vi "Create test signal.vi"(8 "Number of samples":dbl=10000.0, 10 "Downsample factor":i32, 11 "Sample rate":dbl) -> (1 "dt":dbl, 2 "signal out":waveform(dbl)={"t0"=timestamp(0.001 s since 1904-01-01), "dt"=1.0, "Y"=[]}, 3 "Y":fxp<+/-,16,14>[](array[numeric]))   [LabVIEW 2013]
uses:
  <vilib>/measure/NI_MABase.lvlib
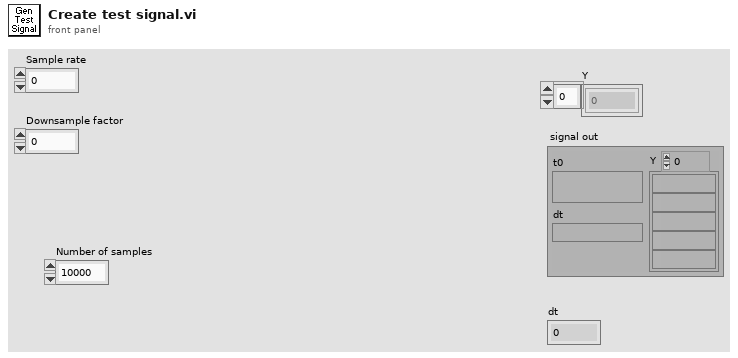
[diagram p1: front panel]
types:
  T1 = cluster{"frequency":dbl, "amplitude":dbl, "phase":dbl}
  T2 = cluster{"frequency":dbl, "amplitude":dbl, "phase":dbl}[]
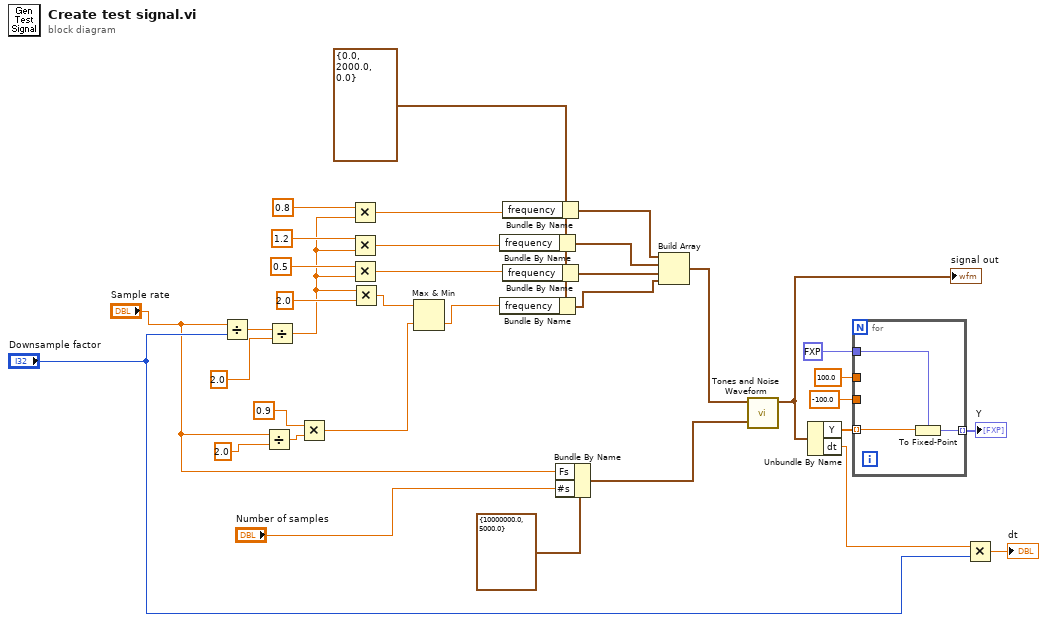
[diagram p0: block diagram]
diagram:
  w20 = T1 {"frequency"=0.0, "amplitude"=2000.0, "phase"=0.0} ("tone f, a, p")
  n1 = Divide(x="Sample rate", y="Downsample factor") -> (x/y=w28:dbl)
  n2 = Divide(x="Sample rate", y=2.0) -> (x/y=w5:dbl)
  n3 = Divide(x=w28, y=2.0) -> (x/y=w22:dbl)
  n4 = Multiply(x=0.9, y=w5) -> (x*y=w2:dbl)
  n5 = Multiply(x=0.8, y=w22) -> (x*y=w21:dbl)
  n6 = Multiply(x=1.2, y=w22) -> (x*y=w19:dbl)
  n7 = Multiply(x=0.5, y=w22) -> (x*y=w18:dbl)
  n8 = Multiply(x=w22, y=2.0 ("x")) -> (x*y=w3:dbl)
  n9 = Max & Min(x=w3, y=w2) -> (min(x,y)=w1:dbl)  [unwired: 1 out]
  n10 = Bundle By Name(cluster=w20, "frequency"=w19) -> (w16:T1)
  n11 = Bundle By Name(cluster=w20, "frequency"=w1) -> (w14:T1)
  n12 = Bundle By Name(cluster=w20, "frequency"=w21) -> (w17:T1)
  n13 = Bundle By Name(cluster=w20, "frequency"=w18) -> (w15:T1)
  n14 = Bundle By Name(cluster=cluster{"Fs":dbl, "#s":dbl} {"Fs"=10000000.0, "#s"=5000.0} ("sampling info"), "Fs"="Sample rate", "#s"="Number of samples") -> (w10:cluster{"Fs":dbl, "#s":dbl})
  n15 = Build Array(w17, w16, w15, w14) -> (w13:T2)
  n16 = call <vilib>:"Tones and Noise Waveform.vi"("sampling info"=w10, "tones"=w13) -> ("signal out"=w32:waveform(dbl))  [unwired: 8 in, 1 out]
  "signal out" <- w32
  n17 = Unbundle By Name(w32) -> ("Y"=w34:dbl[], "dt"=w33:dbl)
  n18 = for {
    tunnel: w34 -> [w36] mode=indexing
    tunnel: fxp<+/-,16,14> 0.0 ("fixed-point type") -> [w38]
    tunnel: [w37] -> w29 mode=indexing
    tunnel: 100.0 -> [_]
    tunnel: -100.0 -> [_]
    n19 = To Fixed-Point(fixed-point type=w38, number=w36) -> (fixed-point=w37:fxp<+/-,16,14>)
  }
  "Y" <- w29
  n20 = Multiply(x=w33, y="Downsample factor") -> (x*y=→"dt":dbl)
